vi "Read Set Button Names.vi"(8 "error in (no error)":errorcluster, 11 "UI Populate Menu in":refnum<class "UI Populate Menu.lvclass">) -> (0 "error out":errorcluster, 2 "Set Button Names":string[](array[string]), 3 "UI Populate Menu out":refnum<class "UI Populate Menu.lvclass">)   [LabVIEW 2011, in "UI Populate Menu.lvclass"]
uses:
  UI Populate Menu.lvclass
  UI Populate Menu.lvclass/UI Populate Menu.ctl
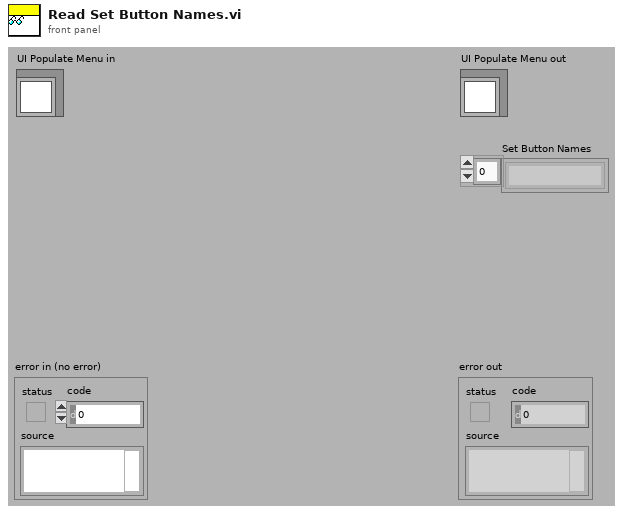
[diagram p1: front panel]
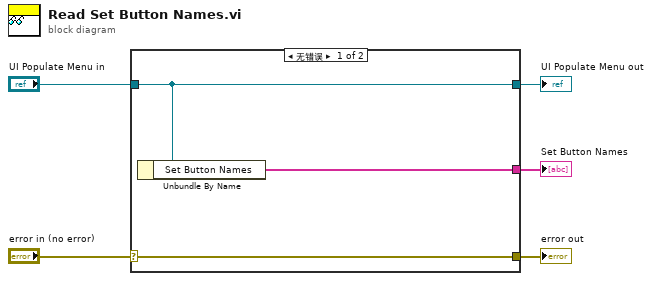
[diagram p0: block diagram]
diagram:
  n1 = case shown="无错误" "error in (no error)" {
    selector: "error in (no error)" -> [w8 w9]
    tunnel: [w8 w9] -> w4
    tunnel: [w7 w10] -> w2
    tunnel: "UI Populate Menu in" -> [w7 w10]
    tunnel: [w6 _] -> w1
    frame No Error {
      n2 = Unbundle By Name(w7) -> ("Set Button Names"=w6:string[])
    }
    frame Error {
    }
  }
  "error out" <- w4
  "UI Populate Menu out" <- w2
  "Set Button Names" <- w1
